vi "ValidateNumInRow.vi"(8 "Number":i32, 9 "Current Cell":T1, 11 "Board":i32[][](array[numeric])) -> (3 "Board":i32[][](array[numeric]), 4 "Valid in Row":bool)   [LabVIEW 2023]
doc: "Checks if Number is Valid in the current Row\n\nInputs\n- Board: Current Board Configuration\n- Row: Row of current Cell\n- Column: Column of current Cell\n- Number: Number to try out in current Cell\n\nOutputs\n- Board: Current Board Configuration\n- Row: Row of current Cell\n- Column: Column of current Cell\n- Number: Number to try out in current Cell\n- Valid in Column: TRUE if Number is valid in current Row"
uses:
  Controls/CurrentCell.ctl
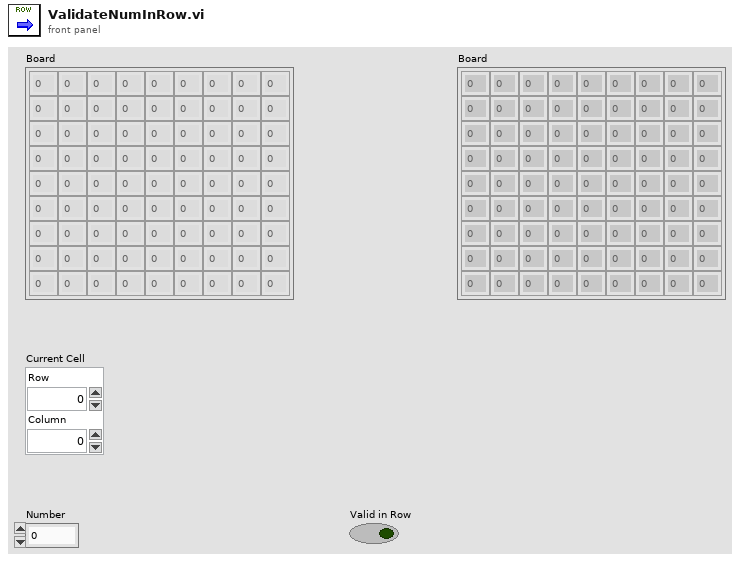
[diagram p1: front panel]
types:
  T1 = typedef "CurrentCell.ctl" = cluster{"Row":i32, "Column":i32}
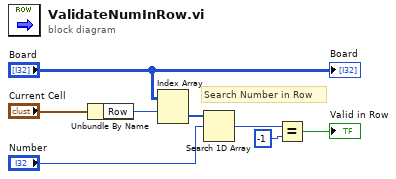
[diagram p0: block diagram]
diagram:
  # "Search Number in Row"
  n1 = Unbundle By Name("Current Cell") -> ("Row"=w3:i32)
  n2 = Index Array(array="Board", index (row)=w3) -> (element=w5:i32[])  [unwired: 1 in]
  n3 = Search 1D Array(1D array=w5, element="Number") -> (index of element=w4:i32)  [unwired: 1 in]
  n4 = Equal?(x=w4, y=-1) -> (x = y?=→"Valid in Row":bool)
  "Board" <- "Board"
